vi "Housekeeping of Plugins.vi"(8 "error in (no error)":errorcluster, 11 "CIFPluginManager in":refnum<class "CIFPluginManager.lvclass">) -> (0 "error out":errorcluster)   [LabVIEW 2021, in "CIFPluginManager.lvclass"]
uses:
  CIFPluginManager.lvclass
  CIFPluginManager.lvclass/CIFPluginManager.ctl
  <vilib>/Utility/miscctls.llb/LVMapReplaceAction.ctl
  <vilib>/CIF Foundation/CIF Utilities/Time/Time_CIF_U.lvlib
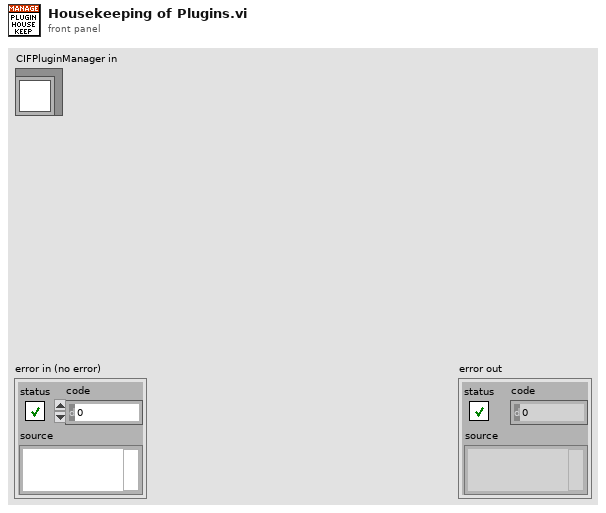
[diagram p1: front panel]
types:
  T1 = typedef "LVMapReplaceAction.ctl" = enum32{"Modify Entry only if found", "Add or Modify Entry", "Delete Entry"}
  T2 = typedef "CIFPluginManager.lvclass/Plugin Management Data Map.ctl" = map{string, T3}
  T3 = typedef "CIFPluginManager.lvclass/Plugin Management Data.ctl" = cluster{"Unique Name":string, "Plugin Type":string, "gRPC Port":i32, "gRPC ID":T4, "Loader Type":T5, "Loader":string, "Version":T6, "Load Timestamp":i64, "Unload Timestamp":i64, "Unloading":bool, "Ready for removal":bool, "status":T7, "channels":T16}
  T4 = typedef "grpc-lvsupport-release.lvlib/grpcId.ctl" = u64
  T5 = typedef "CIFPluginManager.lvclass/Loader Type.ctl" = enum16{"LabVIEW"}
  T6 = typedef "CIFCoreCommon.lvlib/Version.ctl" = cluster{"Major":i32, "Minor":i32, "Fix":i32, "Build":i32}
  T7 = typedef "CIF_Manager_server.lvlib/cif_management_common_PluginStatusData.ctl" = cluster{"state":T8, "timing_statistics":T9, "fifo_statistics":T11, "error":T12, "monitor_doubles":T13, "monitor_u64s":T14, "monitor_i64s":T15}
  T8 = typedef "CIF_Manager_server.lvlib/cif_management_common_PluginStatusData_PluginState.ctl" = enum32{"PLUGINSTATE_UNKNOWN", "PLUGINSTATE_CREATING", "PLUGINSTATE_LISTENING", "PLUGINSTATE_RUNNING", "PLUGINSTATE_CLEANINGUP", "PLUGINSTATE_DESTROYING"}
  T9 = typedef "CIF_Manager_server.lvlib/cif_management_common_TimingStatistics.ctl" = cluster{"period":T10, "wake_error":T10, "execute":T10, "housekeep":T10, "idle":T10, "cleanup":T10, "custom_1":T10, "custom_2":T10}
  T10 = typedef "CIF_Manager_server.lvlib/cif_common_TimingStats.ctl" = cluster{"max":i64, "min":i64, "avg":dbl}
  T11 = typedef "CIF_Manager_server.lvlib/cif_management_common_FifoStatistics.ctl" = cluster{"from_t0":T10, "from_previous_plugin":T10, "output_error":T10}
  T12 = typedef "CIF_Manager_server.lvlib/cif_management_common_Error.ctl" = cluster{"status":bool, "code":i32}
  T13 = typedef "CIF_Manager_server.lvlib/cif_management_common_MonitorDoubles.ctl" = cluster{"double_1":dbl, "double_2":dbl, "double_3":dbl, "double_4":dbl}
  T14 = typedef "CIF_Manager_server.lvlib/cif_management_common_MonitorU64.ctl" = cluster{"u64_1":u64, "u64_2":u64, "u64_3":u64, "u64_4":u64}
  T15 = typedef "CIF_Manager_server.lvlib/cif_management_common_MonitorI64.ctl" = cluster{"i64_1":i64, "i64_2":i64, "i64_3":i64, "i64_4":i64}
  T16 = typedef "CIF_Manager_server.lvlib/cif_management_common_Channels.ctl" = cluster{"channels":T17[]}
  T17 = typedef "CIF_Manager_server.lvlib/cif_management_common_Channel.ctl" = cluster{"name":string, "direction":T18, "type":string, "custom_config":u8[], "connected":bool, "connected_name":string, "forced":bool, "channel_pattern":T19}
  T18 = typedef "CIF_Manager_server.lvlib/cif_management_common_ChannelDirection.ctl" = enum32{"CHANNELDIRECTION_UNKNOWN", "CHANNELDIRECTION_PUBLISHER", "CHANNELDIRECTION_SUBSCRIBER"}
  T19 = typedef "CIF_Manager_server.lvlib/cif_management_common_ChannelPattern.ctl" = enum32{"CHANNELPATTERN_UNKNOWN", "CHANNELPATTERN_TAG", "CHANNELPATTERN_FIFO", "CHANNELPATTERN_MULTIFIFO", "CHANNELPATTERN_BACKPRESSUREFIFO"}
  T20 = typedef "CIFPluginManager.lvclass/Loader Map.ctl" = map{string, T21}
  T21 = typedef "CIFPluginManager.lvclass/Loaders.ctl" = cluster{"Loader Type":T5, "grpc_port":i32, "pid":u32, "gRPC ID":T4, "Load Timestamp":i64, "Unloading":bool, "Ready for removal":bool, "Unload Timestamp":i64}
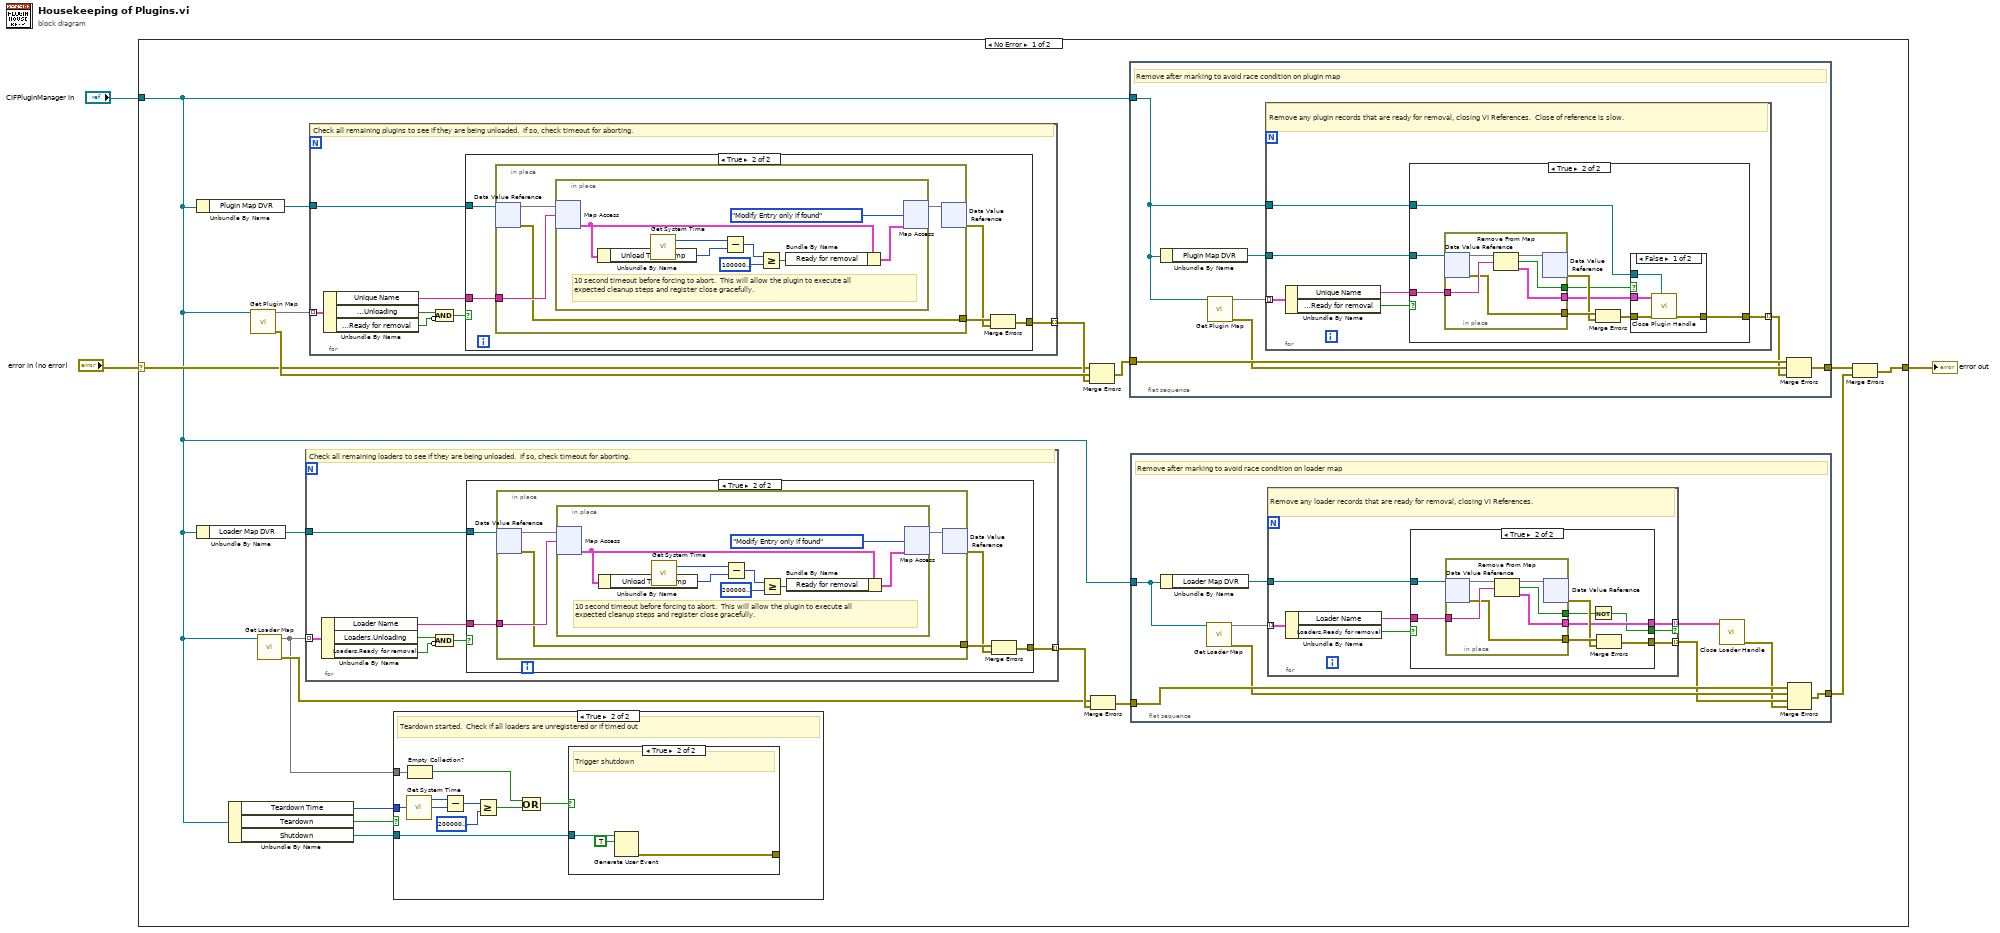
[diagram p0: block diagram]
diagram:
  n1 = case shown="No Error" "error in (no error)" {
    selector: "error in (no error)" -> [w17 w145]
    tunnel: [w9 w145] -> w2
    tunnel: "CIFPluginManager in" -> [w7 _]
    frame No Error {
      n2 = Unbundle By Name(w7) -> ("Plugin Map DVR"=w20:refnum<data-value>)
      n3 = Unbundle By Name(w7) -> ("Loader Map DVR"=w13:refnum<data-value>)
      n4 = Unbundle By Name(w7) -> ("Teardown Time"=w6:i64, "Teardown"=w5:bool, "Shutdown"=w4:refnum<user-event>)
      n5 = call "Get Plugin Map.vi"("CIFPluginManager in"=w7) -> ("error out"=w19:errorcluster, "Plugin Map"=w21:T2)  [unwired: 9 in]
      n6 = call "Get Loader Map.vi"("CIFPluginManager in"=w7) -> ("error out"=w12:errorcluster, "Loader Map"=w8:T20)  [unwired: 9 in]
      n7 = for {
        tunnel: w8 -> [w70] mode=indexing
        tunnel: [w67] -> w14 mode=indexing
        tunnel: w13 -> [w69]
        # "Check all remaining loaders to see if they are being unloaded.  If so, check timeout for aborting."
        n8 = Unbundle By Name(w70) -> ("Loader Name"=w68:string, "Loaders.Unloading"=w66:bool, "Loaders.Ready for removal"=w65:bool)
        n9 = Compound Arithmetic op=AND(w66, invert w65) -> (w64:bool)
        n10 = case shown="True" w64 {
          tunnel: w69 -> [_ w74]
          tunnel: w68 -> [_ w75]
          tunnel: [_ w71] -> w67
          frame False {
          }
          frame True {
            n11 = in-place {
              in-place-border: w75 -> [w79]
              in-place-border: [w76] -> w73
              n12 = in-place-dvr #1(w74) -> (w78:T20, w76:errorcluster)
              n13 = in-place {
                # "10 second timeout before forcing to abort.  This will allow the plugin to execute all expected cleanup steps and register close gracefully."
                n14 = in-place-map #2(w78, w79) -> (w85:T21)  [unwired: 1 in, 1 out]
                n15 = Unbundle By Name(w85) -> ("Unload Timestamp"=w86:i64)
                n16 = call <vilib>:"Get System Time.vi"() -> ("Time (ns)"=w80:i64)  [unwired: 5 in]
                n17 = Subtract(x=w80, y=w86) -> (x-y=w84:i64)
                n18 = Greater Or Equal?(x=w84, y=i64 20000000000) -> (x >= y?=w82:bool)
                n19 = Bundle By Name(cluster=w85, "Ready for removal"=w82) -> (w81:T21)
                n20 = in-place-map #2(w81, LVMapReplaceAction."Modify Entry only if found" ("action")) -> (w77:T20)  [unwired: 2 out]
              }
              n21 = in-place-dvr #1(w77) -> (w72:errorcluster)  [unwired: 1 out]
            }
            n22 = Merge Errors(w73, w72) -> (w71:errorcluster)
          }
        }
      }
      n23 = for {
        tunnel: w21 -> [w127] mode=indexing
        tunnel: [w124] -> w18 mode=indexing
        tunnel: w20 -> [w126]
        # "Check all remaining plugins to see if they are being unloaded.  If so, check timeout for aborting."
        n24 = Unbundle By Name(w127) -> ("Unique Name"=w125:string, "Plugin Management Data.Unloading"=w123:bool, "Plugin Management Data.Ready for removal"=w122:bool)
        n25 = Compound Arithmetic op=AND(w123, invert w122) -> (w121:bool)
        n26 = case shown="True" w121 {
          tunnel: w126 -> [_ w131]
          tunnel: w125 -> [_ w132]
          tunnel: [_ w128] -> w124
          frame False {
          }
          frame True {
            n27 = in-place {
              in-place-border: w132 -> [w136]
              in-place-border: [w133] -> w130
              n28 = in-place-dvr #3(w131) -> (w135:T2, w133:errorcluster)
              n29 = in-place {
                # "10 second timeout before forcing to abort.  This will allow the plugin to execute all expected cleanup steps and register close gracefully."
                n30 = in-place-map #4(w135, w136) -> (w142:T3)  [unwired: 1 in, 1 out]
                n31 = Unbundle By Name(w142) -> ("Unload Timestamp"=w143:i64)
                n32 = call <vilib>:"Get System Time.vi"() -> ("Time (ns)"=w137:i64)  [unwired: 5 in]
                n33 = Subtract(x=w137, y=w143) -> (x-y=w141:i64)
                n34 = Greater Or Equal?(x=w141, y=i64 10000000000) -> (x >= y?=w139:bool)
                n35 = Bundle By Name(cluster=w142, "Ready for removal"=w139) -> (w138:T3)
                n36 = in-place-map #4(w138, LVMapReplaceAction."Modify Entry only if found" ("action")) -> (w134:T2)  [unwired: 2 out]
              }
              n37 = in-place-dvr #3(w134) -> (w129:errorcluster)  [unwired: 1 out]
            }
            n38 = Merge Errors(w130, w129) -> (w128:errorcluster)
          }
        }
      }
      n39 = case shown="True" w5 {
        tunnel: w8 -> [_ w30]
        tunnel: w6 -> [_ w28]
        tunnel: w4 -> [_ w22]
        frame False {
        }
        frame True {
          # "Teardown started.  Check if all loaders are unregistered or if timed out"
          n40 = call <vilib>:"Get System Time.vi"() -> ("Time (ns)"=w29:i64)  [unwired: 5 in]
          n41 = Empty Collection?(1:w30) -> (0:w24:bool)
          n42 = Subtract(x=w29, y=w28) -> (x-y=w26:i64)
          n43 = Greater Or Equal?(x=w26, y=i64 20000000000) -> (x >= y?=w25:bool)
          n44 = Compound Arithmetic op=OR(w24, w25) -> (w23:bool)
          n45 = case shown="True" w23 {
            tunnel: w22 -> [_ w33]
            tunnel: [_ w31] -> _
            frame False {
            }
            frame True {
              # "Trigger shutdown"
              n46 = Generate User Event(user event=w33, event data cluster=TRUE ("event data")) -> (error out=w31:errorcluster)  [unwired: 2 in, 1 out]
            }
          }
        }
      }
      n47 = Merge Errors(w17, w19, w18) -> (w16:errorcluster)
      n48 = Merge Errors(w12, w14) -> (w15:errorcluster)
      n49 = flat-sequence {
        tunnel: [w89] -> w11
        tunnel: w7 -> [w88]
        tunnel: w16 -> [w93]
        frame #0 {
          # "Remove after marking to avoid race condition on plugin map"
          n50 = Unbundle By Name(w88) -> ("Plugin Map DVR"=w94:refnum<data-value>)
          n51 = call "Get Plugin Map.vi"("CIFPluginManager in"=w88) -> ("error out"=w91:errorcluster, "Plugin Map"=w92:T2)  [unwired: 9 in]
          n52 = for {
            tunnel: w92 -> [w100] mode=indexing
            tunnel: [w97] -> w90 mode=indexing
            tunnel: w94 -> [w99]
            tunnel: w88 -> [w96]
            # "Remove any plugin records that are ready for removal, closing VI References.  Close of reference is slow."
            n53 = Unbundle By Name(w100) -> ("Unique Name"=w95:string, "Plugin Management Data.Ready for removal"=w98:bool)
            n54 = case shown="True" w98 {
              tunnel: w99 -> [_ w108]
              tunnel: w95 -> [_ w109]
              tunnel: [_ w104] -> w97
              tunnel: w96 -> [_ w101]
              frame False {
              }
              frame True {
                n55 = in-place {
                  in-place-border: w109 -> [w120]
                  in-place-border: [w118] -> w107
                  in-place-border: [w116] -> w102
                  in-place-border: [w115] -> w103
                  n56 = in-place-dvr #5(w108) -> (w119:T2, w118:errorcluster)
                  n57 = Remove From Map(10:w120, 11:w119) -> (1:w116:T3, 2:w115:bool, 3:w117:T2)
                  n58 = in-place-dvr #5(w117) -> (w106:errorcluster)  [unwired: 1 out]
                }
                n59 = Merge Errors(w107, w106) -> (w105:errorcluster)
                n60 = case shown="False" w103 {
                  tunnel: w105 -> [w113 w114]
                  tunnel: [w112 w114] -> w104
                  tunnel: w102 -> [w111 _]
                  tunnel: w101 -> [w110 _]
                  frame False {
                    n61 = call "Close Plugin Handle.vi"("CIFPluginManager in"=w110, "error in (no error)"=w113, "Plugin Management Data"=w111) -> ("error out"=w112:errorcluster)  [unwired: 8 in]
                  }
                  frame True {
                  }
                }
              }
            }
          }
          n62 = Merge Errors(w93, w91, w90) -> (w89:errorcluster)
        }
      }
      n63 = flat-sequence {
        tunnel: [w40] -> w10
        tunnel: w7 -> [w39]
        tunnel: w15 -> [w41]
        frame #0 {
          # "Remove after marking to avoid race condition on loader map"
          n64 = Unbundle By Name(w39) -> ("Loader Map DVR"=w42:refnum<data-value>)
          n65 = call "Get Loader Map.vi"("CIFPluginManager in"=w39) -> ("error out"=w36:errorcluster, "Loader Map"=w38:T20)  [unwired: 9 in]
          n66 = for {
            tunnel: w38 -> [w49] mode=indexing
            tunnel: [w45] -> w35 mode=indexing
            tunnel: w42 -> [w48]
            tunnel: [w44] -> w37 mode=indexing if=w43
            # "Remove any loader records that are ready for removal, closing VI References."
            n67 = Unbundle By Name(w49) -> ("Loader Name"=w47:string, "Loaders.Ready for removal"=w46:bool)
            n68 = case shown="True" w46 {
              tunnel: w48 -> [_ w56]
              tunnel: w47 -> [_ w57]
              tunnel: [_ w50] -> w45
              tunnel: [_ w53] -> w44
              tunnel: [_ w51] -> w43
              frame False {
              }
              frame True {
                n69 = in-place {
                  in-place-border: w57 -> [w63]
                  in-place-border: [w61] -> w55
                  in-place-border: [w59] -> w53
                  in-place-border: [w58] -> w52
                  n70 = in-place-dvr #6(w56) -> (w62:T20, w61:errorcluster)
                  n71 = Remove From Map(10:w63, 11:w62) -> (1:w59:T21, 2:w58:bool, 3:w60:T20)
                  n72 = in-place-dvr #6(w60) -> (w54:errorcluster)  [unwired: 1 out]
                }
                n73 = Not(x=w52) -> (.not. x?=w51:bool)
                n74 = Merge Errors(w55, w54) -> (w50:errorcluster)
              }
            }
          }
          n75 = call "Close Loader Handle.vi"("Loaders"=w37) -> ("error out"=w34:errorcluster)  [unwired: 10 in]
          n76 = Merge Errors(w41, w36, w35, w34) -> (w40:errorcluster)
        }
      }
      n77 = Merge Errors(w11, w10) -> (w9:errorcluster)
    }
    frame Error {
    }
  }
  "error out" <- w2
